vi "SafeIntakeMode.vi"() -> (1 "Angle Power":dbl, 2 "Roller Power":dbl)   [LabVIEW 2015]
uses:
  Common Code/Intake States.ctl
  Common Code/Intake Commands.ctl
  Robot Global Data.vi
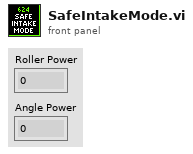
[diagram p1: front panel]
types:
  T1 = typedef "Intake States.ctl" = enum16{"Idle", "Set roller speed", "Move to angle"}
  T2 = typedef "Dashboard Control Data.ctl" = cluster{"Shooter Presets":T3, "Encoder Control":T5, "Steer PID output":cluster{"output high":dbl, "output low":dbl}, " Steer PID gains":cluster{"proportional gain (Kc)":dbl, "integral time (Ti, min)":dbl, "derivative time (Td, min)":dbl}, "Drivetrain Settings":T6, "Vision Packet":T7, "Dashboard Drivetrain Command":T8, "Info/Command Cluster":T10, "Ball Vision Packet":T11, "Intake Presets":T13, "Intake Encoder Control":T15, "Climb Presets":T16}
  T3 = typedef "Shooter Presets.ctl" = cluster{"Batter Shot":T4, "Low Bar Curve Shot":T4, "Deep Middle Shot":T4, "Manual Shot":T4, "Left Ticks Per Rotation":dbl, "Right Ticks Per Rotation":dbl, "Low Bar Shot":T4, "Shooter RPM Tolerance":dbl, "IIR Filter Power":dbl, "Trigger Power":dbl, "Fire from Load Delay":i32, "Angle Pot M":dbl, "Angle Pot B":dbl, "Shooter Deck Length":dbl, "String Pot Dist From Pivot":dbl, "Angle PID gains":cluster{"proportional gain (Kc)":dbl, "integral time (Ti, min)":dbl, "derivative time (Td, min)":dbl}, "Angle Motor Output Range":cluster{"output high":dbl, "output low":dbl}, "Shooter Angle Tolerance":dbl, "Vision Shoot m":dbl, "Vision Shoot b":dbl, "Dist from Axis Cam to Pivot":dbl, "High Goal Center Height":dbl, "Feed Forward Max Accel":dbl, "Feed Forward Kv":dbl, "Backwards Trigger":dbl, "Shot Finish Delay (ms)":dbl, "Angle Max Current":dbl, "Angle Current Trip Time":dbl, "Shooter Intake Angle":dbl}
  T4 = typedef "Shot Presets.ctl" = cluster{"Left Wheel RPM":dbl, "Right Wheel RPM":dbl, "Angle":dbl}
  T5 = typedef "Encoder Control.ctl" = cluster{"Right Tick Constant":dbl, "Left Tick Constant":dbl, "Reset?":bool, "Y Dist":cluster{"PID gains":cluster{"proportional gain (Kc)":dbl, "integral time (Ti, min)":dbl, "derivative time (Td, min)":dbl}}, "Y Stop Thresh":dbl, "Y Stop Speed":dbl}
  T6 = typedef "Drivetrain Settings.ctl" = cluster{"Gyro Tolerance":dbl, "Throttle Ramp (ms)":dbl, "Angular rate compensation":bool, "Throttle to Rate Scale":dbl, "Rate compensation gain":dbl, "Kv":dbl, "Ka":dbl, "Feed Forward P":dbl, "Feed Forward D":dbl}
  T7 = typedef "Goal Vision Packet.ctl" = cluster{"Distance":dbl, "Center X":dbl, "Center Y":dbl, "Found Target?":bool}
  T8 = typedef "Dashboard Drivetrain Command.ctl" = cluster{"Drivetrain Vision":T9, "Vision Scale Down Speed":dbl, "Goal Vision PID gains":cluster{"proportional gain (Kc)":dbl, "integral time (Ti, min)":dbl, "derivative time (Td, min)":dbl}, "Ball Vision PID gains":cluster{"proportional gain (Kc)":dbl, "integral time (Ti, min)":dbl, "derivative time (Td, min)":dbl}}
  T9 = typedef "Drivetrain Vision.ctl" = cluster{"Goal Window":dbl, "Ball Window":dbl}
  T10 = typedef "Ball Tracking Command Cluster.ctl" = cluster{"Distance to Ball":dbl, "Desired Angle":dbl, "Command":enum16{"Turn to Ball", "Turn to Angle", "Get Distance"}, "Pixels from Center":dbl}
  T11 = typedef "Ball Vision Packet.ctl" = cluster{"Ball Detected?":bool, "Distance to Ball":dbl, "Desired Angle":dbl, "Pixels from Center":dbl, "Tracking mode":T12}
  T12 = typedef "Tracking Mode.ctl" = enum16{"Turn to Ball", "Turn to Angle"}
  T13 = typedef "Intake Presets.ctl" = cluster{"Intake Speed":dbl, "Outake Speed":dbl, "Low Height":dbl, "High Height":dbl, "Full Height":dbl, "Angle Speed":dbl, "Fast Angle":dbl, "Encoder Scale Factor":dbl, "Load Height":dbl, "Output Range":T14, "PID Params":cluster{"PID gains":cluster{"proportional gain (Kc)":dbl, "integral time (Ti, min)":dbl, "derivative time (Td, min)":dbl}}, "Rotation Power Max/Min":dbl, "MaxCurrent":dbl, "Intake Trip Time":dbl, "FeedForwardMaxAcceleration":dbl, "FeedForwardMaxVelocity":dbl, "Ka":dbl, "Kw":dbl, "AngleTolerance":dbl}
  T14 = typedef "Drivetrain Output Range.ctl" = cluster{"output high":dbl, "output low":dbl}
  T15 = typedef "IntakeEcoderControl.ctl" = cluster{"Arm Tick Constant":dbl, "Reset?":bool, "Y Dist":cluster{"PID gains":cluster{"proportional gain (Kc)":dbl, "integral time (Ti, min)":dbl, "derivative time (Td, min)":dbl}}, "Y Stop Thresh":dbl, "Y Stop Speed":dbl}
  T16 = typedef "Climb Presets.ctl" = cluster{"Pull Power":dbl, "Unpin Power":dbl, "Time to Hold":dbl}
  T17 = typedef "Intake Commands Cluster.ctl" = cluster{"Intake Commands":T18, "Intake Mode":T19, "Encoder Constraint":dbl}
  T18 = typedef "Intake Commands.ctl" = enum16{"Unload", "Load", "Pull up", "Drop low", "Idle", "Lift Half"}
  T19 = typedef "Intake Mode.ctl" = enum16{"Safe", "Auto", "Manual"}
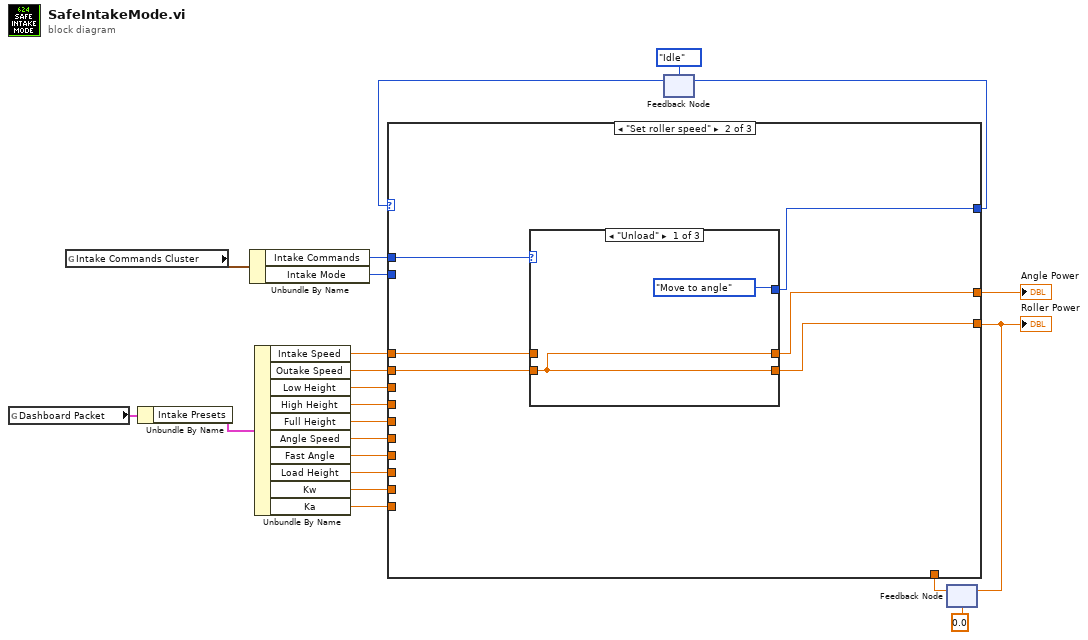
[diagram p0: block diagram]
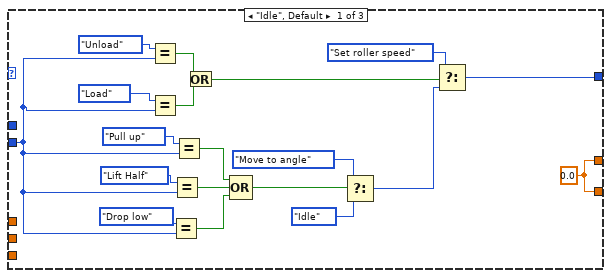
[diagram p2: hidden frame]
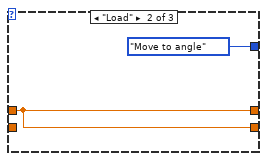
[diagram p3: hidden frame]
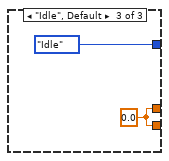
[diagram p4: hidden frame]
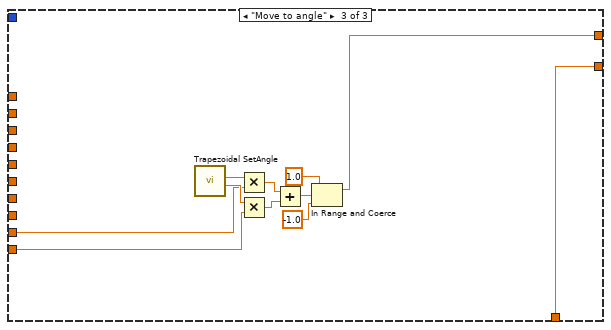
[diagram p5: hidden frame]
diagram:
  n1 = global read "Robot Global Data.vi" "Dashboard Packet"() -> (w22:T2)
  n2 = global read "Robot Global Data.vi" "Intake Commands Cluster"() -> (w8:T17)
  n3 = Unbundle By Name(w22) -> ("Intake Presets"=w21:T13)
  n4 = Unbundle By Name(w8) -> ("Intake Commands"=w13:T18, "Intake Mode"=w1:T19)
  n5 = Unbundle By Name(w21) -> ("Intake Speed"=w20:dbl, "Outake Speed"=w19:dbl, "Low Height"=w18:dbl, "High Height"=w17:dbl, "Full Height"=w16:dbl, "Angle Speed"=w15:dbl, "Fast Angle"=w14:dbl, "Load Height"=w7:dbl, "Kw"=w3:dbl, "Ka"=w2:dbl)
  n6 = feedback #1(Intake_States."Idle" ("Intake States")) -> (w12:T1)
  n7 = feedback #2(0.0 ("Intake Speed")) -> (w9:dbl)
  n8 = case shown="\"Set roller speed\"" w12 {
    tunnel: w20 -> [_ w47 _]
    tunnel: w19 -> [_ w46 _]
    tunnel: w18 -> [_ _ _]
    tunnel: w17 -> [_ _ _]
    tunnel: w16 -> [_ _ _]
    tunnel: w15 -> [_ _ _]
    tunnel: w14 -> [_ _ _]
    tunnel: w13 -> [_ w43 _]
    tunnel: [w25 w44 _] -> w11
    tunnel: [w24 w45 w64] -> w5
    tunnel: w9 -> [_ _ w64]
    tunnel: w7 -> [_ _ _]
    tunnel: [w24 w42 w54] -> w6
    tunnel: w3 -> [_ _ w61]
    tunnel: w2 -> [_ _ w60]
    tunnel: w1 -> [w23 _ _]
    frame "Idle", Default {
      w24 = 0.0
      n9 = Equal?(x=Intake_Commands."Unload" ("Intake Commands"), y=w23) -> (x = y?=w39:bool)
      n10 = Equal?(x=Intake_Commands."Load" ("Intake Commands"), y=w23) -> (x = y?=w38:bool)
      n11 = Equal?(x=Intake_Commands."Drop low" ("Intake Commands"), y=w23) -> (x = y?=w32:bool)
      n12 = Equal?(x=Intake_Commands."Lift Half" ("Intake Commands"), y=w23) -> (x = y?=w33:bool)
      n13 = Equal?(x=Intake_Commands."Pull up" ("Intake Commands"), y=w23) -> (x = y?=w34:bool)
      n14 = Or(x=w39, y=w38) -> (x .or. y?=w31:bool)
      n15 = Compound Arithmetic op=OR(w34, w33, w32) -> (w29:bool)
      n16 = Select(t=Intake_States."Move to angle" ("Intake States"), s=w29, f=Intake_States."Idle" ("Intake States")) -> (s? t:f=w26:T1)
      n17 = Select(t=Intake_States."Set roller speed" ("Intake States"), s=w31, f=w26) -> (s? t:f=w25:T1)
    }
    frame "Set roller speed" {
      n18 = case shown="\"Unload\"" w43 {
        tunnel: w47 -> [_ w50 _]
        tunnel: w46 -> [w48 _ _]
        tunnel: [w48 w50 w52] -> w45
        tunnel: [Intake_States."Move to angle" ("Intake States") Intake_States."Move to angle" ("Intake States") Intake_States."Idle" ("Intake States")] -> w44
        tunnel: [w48 w50 w52] -> w42
        frame "Unload" {
        }
        frame "Load" {
        }
        frame "Idle", Default {
          w52 = 0.0 ("Intake Speed")
        }
      }
    }
    frame "Move to angle" {
      n19 = call "Trapezoidal SetAngle.vi"() -> ("Angular Acceleration"=w62:dbl, "Angular Velocity"=w63:dbl)  [unwired: 8 in, 2 out]
      n20 = Multiply(x=w63, y=w61) -> (x*y=w58:dbl)
      n21 = Multiply(x=w62, y=w60) -> (x*y=w59:dbl)
      n22 = Add(x=w58, y=w59) -> (x+y=w57:dbl)
      n23 = In Range and Coerce(upper limit=1.0, x=w57, lower limit=-1.0) -> (coerced(x)=w54:dbl)  [unwired: 1 out]
    }
  }
  "Angle Power" <- w6
  "Roller Power" <- w5
  n24 = feedback-in #1(w11) -> ()
  n25 = feedback-in #2(w5) -> ()
